vi "PQlistAndCreateColumns.vi"(6 "column type":string, 8 "error in":errorcluster, 9 "table":string[](array[string]), 10 "table name":string, 11 "conn":u64) -> (0 "error out":errorcluster, 3 "conn_out":u64)   [LabVIEW 2019, in "libpqutility64.lvlib"]
uses:
  libpqutility64.lvlib
  libpqlv64/src/PQresultErrorMessage.vi
  PQclear.vi
  libpqlv64/src/PQsendQuery.vi
  libpqlv64/src/PQgetResult.vi
  libpqlv64/src/PQresultStatus.vi
  PQgetColumn.vi
  libpqlv64/src/PQclear.vi
  PQfetchTables.vi
  libpqlv64/src/PQgetvalue.vi
  libpqlv64/src/PQntuples.vi
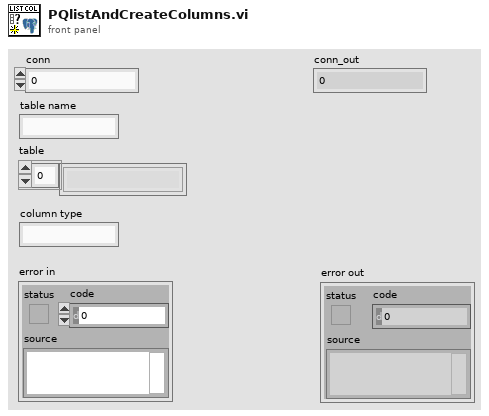
[diagram p1: front panel]
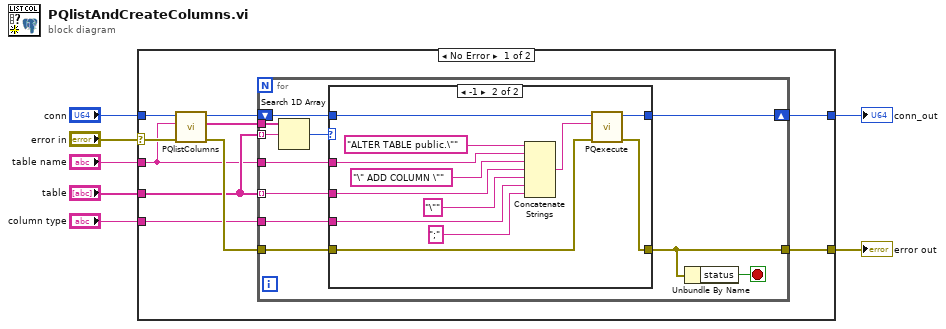
[diagram p0: block diagram]
diagram:
  n1 = case shown="No Error" "error in" {
    selector: "error in" -> [w16 w44]
    tunnel: "conn" -> [w17 w43]
    tunnel: [w10 w43] -> w5
    tunnel: "table" -> [w9 _]
    tunnel: [w13 w44] -> w4
    tunnel: "table name" -> [w8 _]
    tunnel: "column type" -> [w12 _]
    frame No Error {
      n2 = call "PQlistColumns.vi"("error in"=w16, "table"=w8, "conn"=w17) -> ("error out"=w14:errorcluster, "Data"=w15:string[], "conn_out"=w11:u64)  [unwired: 6 in]
      n3 = for {
        tunnel: w15 -> [w20]
        tunnel: w9 -> [w19] mode=indexing
        tunnel: w8 -> [w26]
        tunnel: w9 -> [w27] mode=indexing
        tunnel: [w25] -> w13
        tunnel: w14 -> [w23]
        tunnel: w12 -> [w22]
        shift-right: [w21] -> w10
        shift-left: w11 -> [w24]
        stop <- w28 stop-if-true
        n4 = Search 1D Array(1D array=w20, element=w19) -> (index of element=w18:i32)  [unwired: 1 in]
        n5 = case shown="-1" w18 {
          tunnel: w26 -> [_ w39]
          tunnel: w27 -> [_ w37]
          tunnel: [w30 w40] -> w25
          tunnel: w24 -> [w29 w36]
          tunnel: w23 -> [w30 w35]
          tunnel: w22 -> [_ w32]
          tunnel: [w29 w34] -> w21
          frame 0, Default {
          }
          frame -1 {
            n6 = Concatenate Strings("ALTER TABLE public.\"", w39, "\" ADD COLUMN \"", w37, "\"" ("string"), w32, ";") -> (w41:string)
            n7 = call "PQexecute.vi"("error in"=w35, "SQL querry"=w41, "conn"=w36) -> ("error out"=w40:errorcluster, "conn_out"=w34:u64)  [unwired: 7 in]
          }
        }
        n8 = Unbundle By Name(w25) -> ("status"=w28:bool)
      }
    }
    frame Error {
    }
  }
  "conn_out" <- w5
  "error out" <- w4
